vi "Test Get Aggregated Code Coverage Ignores Framework.vi"(8 "error in (no error)":errorcluster, 11 "Test Case In":refnum<class "Coverage Test.lvclass">) -> (0 "error out":errorcluster, 3 "Test Case Out":refnum<class "Coverage Test.lvclass">)   [LabVIEW 2020, in "LUnit Tests.lvlib" / "Coverage Test.lvclass"]
uses:
  Coverage Test.lvclass
  C:/Program Files (x86)/National Instruments/LabVIEW 2020/vi.lib/Astemes/LUnit/Test Case.lvclass
  source/Framework/Coverage Analyzer/Coverage Analyzer.lvclass
  <vilib>/Astemes/LUnit/Test Case.lvclass/Test Case.ctl
  <vilib>/Astemes/LUnit/LUnit Assertion Result.lvclass/LUnit Assertion Result.ctl
  <vilib>/Astemes/LUnit/LUnit Test Case Result.lvclass/LUnit Test Case Result.ctl
  <vilib>/Astemes/LUnit/LUnit Method Result.lvclass/LUnit Method Result.ctl
  01074fa8-ee8a-411d-bc8b-fc92c4f90959.vi
  <vilib>/Astemes/LUnit/Palette/Pass.vi
  <vilib>/Astemes/LUnit/Palette/Fail.vi
  <vilib>/Astemes/LUnit/Compare Variants.vi
  <vilib>/Astemes/LUnit/Describe Comparison.vi
  <vilib>/Astemes/LUnit/Set Assertion Type.vi
  <vilib>/Astemes/LUnit/Add test result.vi
  <vilib>/Astemes/LUnit/LUnit Write Passed.vi
  <vilib>/Astemes/LUnit/LUnit Write Message.vi
  <vilib>/Astemes/LUnit/LUnit Write Description.vi
  <vilib>/Astemes/LUnit/Variant to string.vi
  <vilib>/Astemes/LUnit/LUnit Write Assertion Type.vi
  <vilib>/Astemes/LUnit/LUnit Record Assertion Result.vi
  <vilib>/Astemes/LUnit/LUnit Aggregate Assertion Results.vi
  <vilib>/Astemes/LUnit/Assertion Result/LUnit Read Status.vi
  <vilib>/Astemes/LUnit/LUnit Read Message.vi
  <vilib>/Astemes/LUnit/LUnit Read Description.vi
  <vilib>/Astemes/LUnit/Method Result/LUnit Merge Status.vi
  <vilib>/Astemes/LUnit/LUnit Concatenate result strings.vi
  <vilib>/Utility/Data Type/Get Type Information.vi
  <vilib>/Utility/LVClass/Get LV Class Name.vi
  <vilib>/Astemes/LUnit/LUnit Assertion Result.lvclass
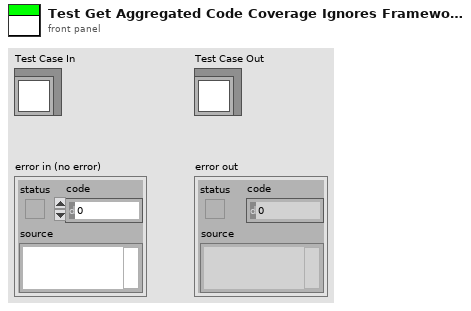
[diagram p1: front panel]
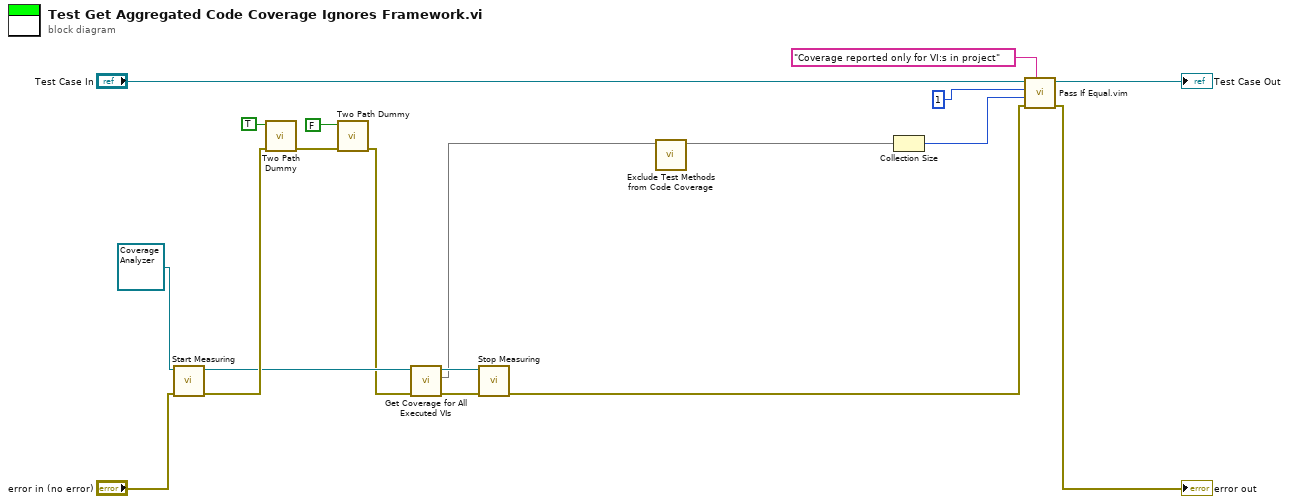
[diagram p0: block diagram]
diagram:
  n1 = call "Start Measuring.vi"("error in (no error)"="error in (no error)", "Coverage Analyzer in"=refnum<class "Coverage Analyzer.lvclass"> refnum) -> ("error out"=w12:errorcluster, "Coverage Analyzer out"=w7:refnum<class "Coverage Analyzer.lvclass">)  [unwired: 8 in]
  n2 = call "Two Path Dummy.vi"("error in (no error)"=w12, "Boolean"=TRUE) -> ("error out"=w16:errorcluster)  [unwired: 9 in]
  n3 = call "Two Path Dummy.vi"("error in (no error)"=w16, "Boolean"=FALSE) -> ("error out"=w5:errorcluster)  [unwired: 9 in]
  n4 = call "Get Coverage for All Executed VIs.vi"("error in (no error)"=w5, "Coverage Analyzer in"=w7) -> ("error out"=w8:errorcluster, "Code Coverage"=w3:map{path, dbl}, "Coverage Analyzer out"=w6:refnum<class "Coverage Analyzer.lvclass">)  [unwired: 7 in]
  n5 = call "Stop Measuring.vi"("error in (no error)"=w8, "Coverage Analyzer in"=w6) -> ("error out"=w10:errorcluster)  [unwired: 8 in, 1 out]
  n6 = call "Exclude Test Methods from Code Coverage.vi"("Code Coverage"=w3) -> ("Filtered Code Coverage"=w2:map{path, dbl})  [unwired: 10 in]
  n7 = Collection Size(1:w2) -> (0:w1:i32)
  n8 = call "Pass If Equal.vim"("Description"="Coverage reported only for VI:s in project", "error in (no error)"=w10, "Actual"=w1, "Expected"=1 ("size"), "LUnit Test Case In"="Test Case In") -> ("error out"=→"error out":errorcluster, "LUnit Test Case Out"=→"Test Case Out":refnum<class "Coverage Test.lvclass">)  [unwired: 5 in]
